vi "Get_A_and_Shift.vi"() -> ()   [LabVIEW 2010]
panel:
  in  "Frequency":dbl
  out "Amplitude":dbl
  out "Shift":dbl
  out "error out":errorcluster
  in  "error in (no error)":errorcluster
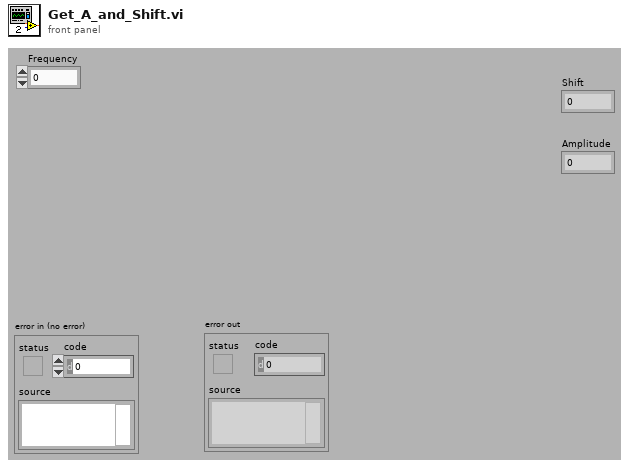
[diagram p1: front panel]
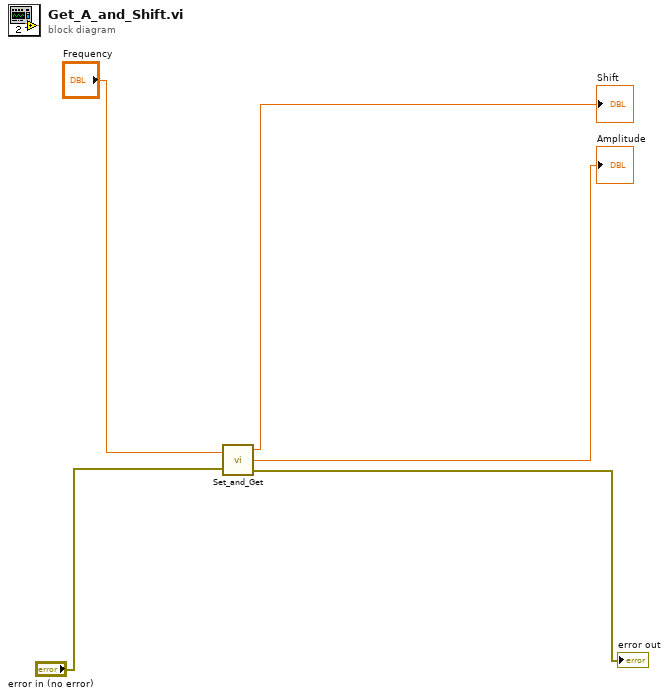
[diagram p0: block diagram]
diagram:
  n1 = call "Set_and_Get.vi"("error in (no error)"="error in (no error)", "Frequency"="Frequency") -> ("error out"=→"error out":errorcluster, "Amplitude"=→"Amplitude":dbl, "Phase Shift"=→"Shift":dbl)
